vi "DSF.Engine.Transfer.Offset Inline Buffer.vi"(8 "error in (no error)":errorcluster, 9 "group engine offset":u64, 10 "Engine Pointer":refnum<class "Memory.Pointer.lvclass">, 11 "Transfer in":refnum<class "DSF.Engine.Transfer.lvclass">) -> (0 "error out":errorcluster, 3 "Transfer out":refnum<class "DSF.Engine.Transfer.lvclass">)   [LabVIEW 2017, in "DSF.Engine.lvlib" / "DSF.Engine.Transfer.lvclass"]
uses:
  DSF.Engine.Transfer.lvclass
  <vilib>/NI/Memory Manager/Classes/Pointer/Memory.Pointer.lvclass
  DSF.Engine.Transfer.lvclass/DSF.Engine.Transfer.ctl
  Pointer/DSF.Engine.Pointer.DBL.lvclass
  C:/Program Files (x86)/National Instruments/LabVIEW 2017/vi.lib/NI/Memory Manager/Classes/Pointer/Memory.Pointer.lvclass
  <vilib>/NI/Memory Manager/Classes/Pointer/Memory.Pointer.lvclass/Memory.Pointer.ctl
  <vilib>/NI/Memory Manager/Classes/Pointer/Memory.Pointer.Parameter Check.Subset.vi
  <vilib>/NI/Memory Manager/Classes/Pointer/Memory.Pointer.Get Address.vi
  <vilib>/NI/Memory Manager/Classes/Pointer/Memory.Pointer.Encapsulate.vi
  <vilib>/NI/Memory Manager/Classes/Pointer/Memory.Pointer.Parameter Check.Null Pointer.vi
  <vilib>/NI/Memory Manager/Classes/Pointer/Memory.Pointer.Errors.vi
  <vilib>/NI/Memory Manager/Classes/Pointer/Memory.Pointer.Errors.Out of Bounds.vi
  <vilib>/NI/Memory Manager/Classes/Pointer/Memory.Pointer.Get Size.vi
  <vilib>/NI/Memory Manager/Classes/Pointer/Memory.Pointer.Set Size.vi
  <vilib>/NI/Memory Manager/Classes/Pointer/Memory.Pointer.Set Address.vi
  <vilib>/NI/Memory Manager/Classes/Pointer/Memory.Pointer.Set Allocated.vi
  <vilib>/NI/Memory Manager/Classes/Pointer/Memory.Pointer.Errors.Null Pointer.vi
  <vilib>/NI/Memory Manager/VIs/Source.Write.String.vi
  <vilib>/NI/Memory Manager/Classes/Pointer/Memory.Pointer.Errors.Write Pointer Size.vi
  <vilib>/NI/Memory Manager/Classes/Pointer/Memory.Pointer.Errors.Create Error.vi
  <vilib>/NI/Memory Manager/VIs/Source.Write.Scalar.Base10.vi
  <vilib>/NI/Memory Manager/VIs/Source.Write.Scalar.Base10 (U64).vi
  <vilib>/NI/Memory Manager/VIs/New Error Cluster Constant.vi
  <vilib>/NI/Memory Manager/VIs/New Error Cluster Constant (512B).vi
  <vilib>/NI/Memory Manager/VIs/Error Cluster.Set Status.vi
  <vilib>/NI/Memory Manager/VIs/Error Cluster.Set Code.vi
  <vilib>/NI/Memory Manager/VIs/Error Cluster.Set VI Source.vi
  <vilib>/NI/Memory Manager/Constants/Memory.Constants.vi
  <vilib>/NI/Memory Manager/Constants/Memory.Constants.Library Name.vi
  <vilib>/NI/Memory Manager/Classes/Pointer/Memory.Pointer.Errors.Get Info.vi
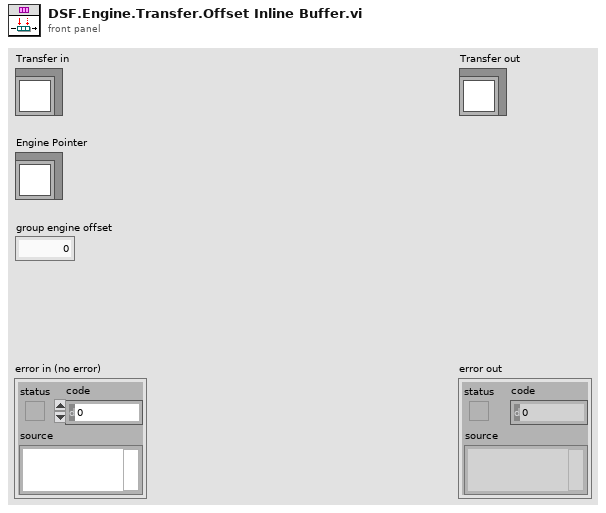
[diagram p1: front panel]
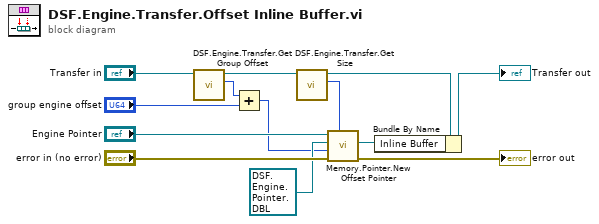
[diagram p0: block diagram]
diagram:
  n1 = call "DSF.Engine.Transfer.Get Group Offset.vi"("Transfer in"="Transfer in") -> ("group offset"=w9:u64, "Transfer out"=w7:refnum<class "DSF.Engine.Transfer.lvclass">)  [unwired: 9 in]
  n2 = Add(x=w9, y="group engine offset") -> (x+y=w1:u64)
  n3 = call "DSF.Engine.Transfer.Get Size.vi"("Transfer in"=w7) -> ("size"=w2:u64, "Transfer out"=w6:refnum<class "DSF.Engine.Transfer.lvclass">)  [unwired: 9 in]
  n4 = call <vilib>:"Memory.Pointer.New Offset Pointer.vi"("length (-1: rest)"=w2, "error in (no error)"="error in (no error)", "offset (0)"=w1, "offset Pointer type"=refnum<class "DSF.Engine.Pointer.DBL.lvclass"> refnum ("Inline Buffer"), "base Pointer in"="Engine Pointer") -> ("error out"=→"error out":errorcluster, "offset Pointer"=w3:refnum<class "DSF.Engine.Pointer.DBL.lvclass">)  [unwired: 3 in, 2 out]
  n5 = Bundle By Name(cluster=w6, "Inline Buffer"=w3) -> (→"Transfer out":refnum<class "DSF.Engine.Transfer.lvclass">)
